vi "PI_TWC.vi"(0 "System no.":i32=1, 5 "error in":errorcluster) -> (19 "error out":errorcluster)   [LabVIEW 8.6]
doc: "Clears the trigger wave settings for the waveform.\n\nValid for E-710"
panel:
  # "Clears the trigger wave settings for the waveform."
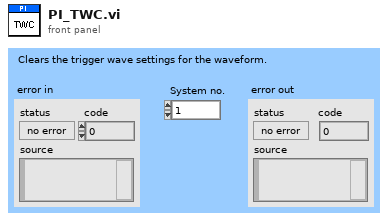
[diagram p1: front panel]
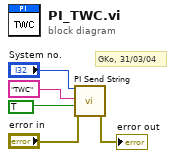
[diagram p0: block diagram]
diagram:
  # "GKo, 31/03/04"
  n1 = call "PI Send String.vi"("System no."="System no.", "String to send"="TWC", "Attach Linefeed?"=TRUE, "error in"="error in") -> ("error out"=→"error out":errorcluster)  [unwired: 15 out]
